vi "strings.vi"() -> ()   [LabVIEW 2022 SP3]
panel:
  in  "Label Contents":dbl
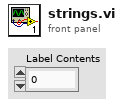
[diagram p1: front panel]
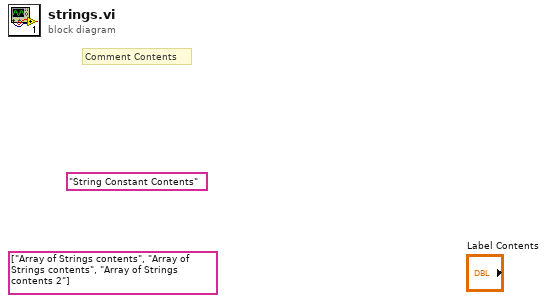
[diagram p0: block diagram]
diagram:
  (unwired) string[] ["Array of Strings contents", "Array of Strings contents", "Array of Strings contents 2"]
  (unwired) "String Constant Contents"
  # "Comment Contents"
